vi "ExcelDispatchAutoDetect.vi"() -> ()   [LabVIEW 2012]
panel:
  in  "stop":bool
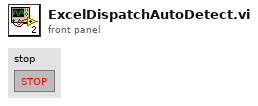
[diagram p1: front panel]
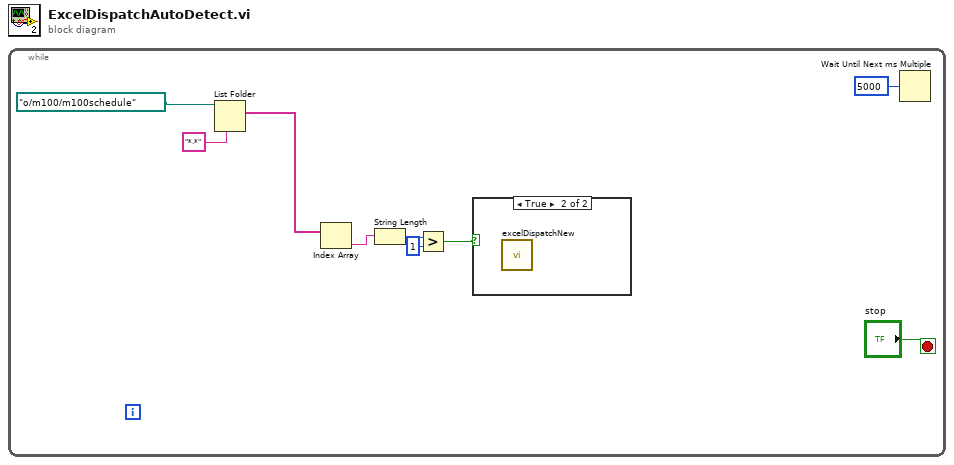
[diagram p0: block diagram]
diagram:
  n1 = while {
    stop <- "stop" stop-if-true
    n2 = List Folder(path=path "o:/m100/m100schedule" ("path (use dialog)"), pattern="*.*") -> (filenames=w5:string[])  [unwired: 2 in, 3 out]
    n3 = Index Array(array=w5) -> (element=w4:string)  [unwired: 1 in]
    n4 = String Length(string=w4) -> (length=w3:i32)
    n5 = Greater?(x=w3, y=1) -> (0:w1:bool)
    n6 = case shown="True" w1 {
      frame False {
      }
      frame True {
        n7 = call "excelDispatchNew.vi"() -> ()  [unwired: 12 in]
      }
    }
    n8 = Wait Until Next ms Multiple(millisecond multiple=u32 5000) -> ()  [unwired: 1 out]
  }
